vi "BuildInsertQuery.vi"(8 "error in (no error)":errorcluster, 10 "QueryBuilderData":T1) -> (0 "error out":errorcluster, 2 "Query":string)   [LabVIEW 2020]
uses:
  DataTypes/QuiryBuilderData--Cluster.ctl
panel:
  in  "CommandText":string="INSERT INTO [BRS].[dbo].[Inventory] (Stocker_ID,Module_no,Column_no,Row_no,Location_Status) VALUES (C,29,1,1,1)"
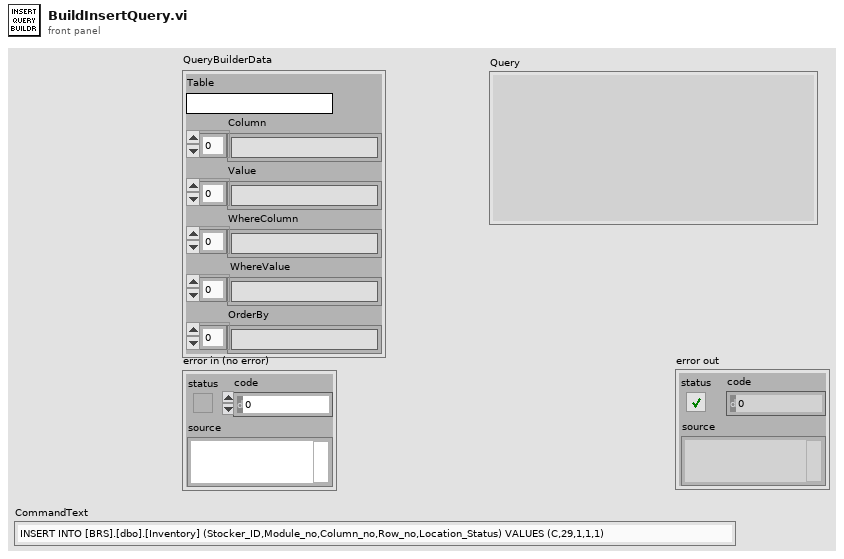
[diagram p1: front panel]
types:
  T1 = typedef "QuiryBuilderData--Cluster.ctl" = cluster{"Table":string, "Column":string[], "Value":string[], "WhereColumn":string[], "WhereValue":string[], "OrderBy":string[]}
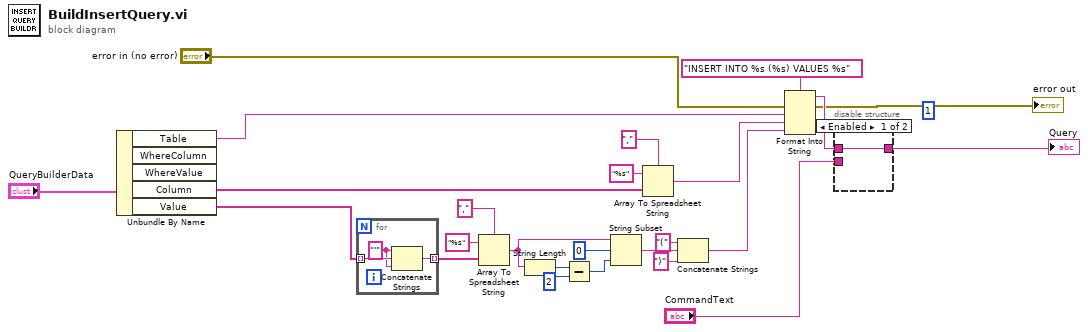
[diagram p0: block diagram]
diagram:
  (unwired) 1 ("Options")
  n1 = Unbundle By Name("QueryBuilderData") -> ("Table"=w3:string, "Column"=w5:string[], "Value"=w4:string[])  [unwired: 2 out]
  n2 = for {
    tunnel: w4 -> [w28] mode=indexing
    tunnel: [w26] -> w17 mode=indexing
    w27 = "'" ("string")
    n3 = Concatenate Strings(w27, w28, w27) -> (w26:string)
  }
  n4 = Array To Spreadsheet String(delimiter (Tab)=",", array=w17, 3:"%s" ("format string")) -> (spreadsheet string=w14:string)
  n5 = String Length(string=w14) -> (length=w12:i32)
  n6 = Subtract(x=w12, y=2) -> (x-y=w9:i32)
  n7 = String Subset(string=w14, offset (0)=0, length (rest)=w9) -> (substring=w10:string)
  n8 = Array To Spreadsheet String(delimiter (Tab)=",", array=w5, 3:"%s" ("format string")) -> (spreadsheet string=w21:string)
  n9 = Concatenate Strings("(" ("string"), w10, ")" ("string")) -> (w8:string)
  n10 = Format Into String(format string="INSERT INTO %s (%s) VALUES %s", error in="error in (no error)", w3, w21, w8) -> (resulting string=w7:string, error out=→"error out":errorcluster)  [unwired: 1 in]
  n11 = disable-structure shown="Enabled" {
    disable-tunnel: w7 -> [w29 _]
    disable-tunnel: [w29 w30] -> w1
    disable-tunnel: "CommandText" -> [_ w30]
    frame Enabled {
    }
    frame Disabled {
    }
  }
  "Query" <- w1
